vi "Wait on Read Loop.vi"(8 "error in (no error)":errorcluster, 10 "Value":bool, 11 "Terminal in":refnum<class "Terminal.lvclass">) -> (0 "error out":errorcluster, 1 "Timed Out?":bool, 3 "Terminal out":refnum<class "Terminal.lvclass">)   [LabVIEW 2020, in "Terminal.lvlib" / "Terminal.lvclass"]
uses:
  Terminal.lvclass
  Terminal.lvclass/Terminal.ctl
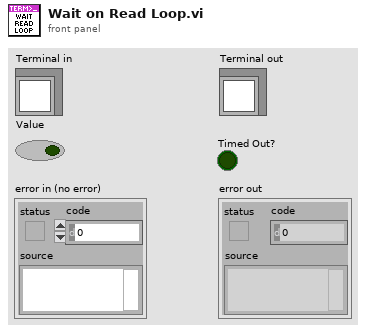
[diagram p1: front panel]
types:
  T1 = typedef "Terminal.lvlib/Terminal.lvclass/Ref Data.ctl" = cluster{"Connection":refnum<class "Connection.lvclass">, "Read Loop Running":bool, "Parse State":T2, "Terminal Options":T7, "Font Metrics":T10, "Scroll":i32, "Close Read Loop":bool}
  T2 = typedef "Terminal.lvlib/Terminal.lvclass/Parse State.ctl" = cluster{"Buffer State":T3, "Cursor":T4, "Attributes":T6}
  T3 = typedef "Terminal.lvlib/Terminal.lvclass/Buffer State.ctl" = cluster{"Sequence":string, "ESC":bool, "Alt Buf":bool}
  T4 = typedef "Terminal.lvlib/Terminal.lvclass/Cursor.ctl" = cluster{"Cur":T5, "Saved":T5}
  T5 = typedef "Terminal.lvlib/Terminal.lvclass/Position.ctl" = cluster{"Row":i32, "Col":i32}
  T6 = typedef "Terminal.lvlib/Text Attributes.ctl" = cluster{"FG":u32, "BG":u32, "Bold":bool, "Italic":bool, "Underline":bool, "Strike":bool, "Inverse":bool}
  T7 = typedef "Terminal.lvlib/Terminal Options.ctl" = cluster{"Implied CR with LF":bool, "Local Echo":bool, "Tab Width":i32, "Color Scheme":T8, "Default FG":T9, "Default BG":T9, "History Length":i32, "Font Face":string, "Font Size":i16, "Rows":i32, "Cols":i32}
  T8 = typedef "Terminal.lvlib/Color Scheme.ctl" = cluster{"Black":u32, "Red":u32, "Green":u32, "Yellow":u32, "Blue":u32, "Magenta":u32, "Cyan":u32, "White":u32, "Bright Black":u32, "Bright Red":u32, "Bright Green":u32, "Bright Yellow":u32, "Bright Blue":u32, "Bright Magenta":u32, "Bright Cyan":u32, "Bright White":u32}
  T9 = typedef "Terminal.lvlib/Color.ctl" = i8
  T10 = typedef "Terminal.lvlib/Terminal.lvclass/Font Metrics.ctl" = cluster{"Width":i16, "Height":i16}
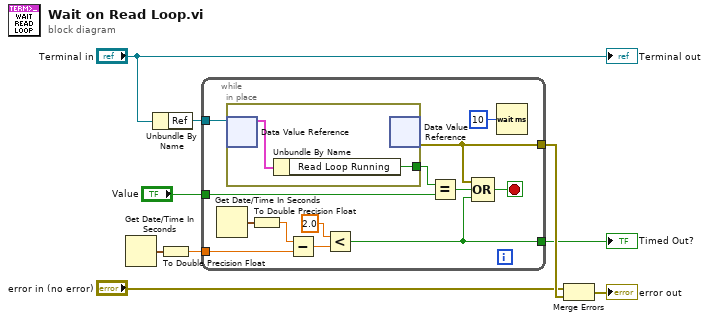
[diagram p0: block diagram]
diagram:
  n1 = Get Date/Time In Seconds() -> (seconds since 1Jan1904=w4:timestamp)
  n2 = Unbundle By Name("Terminal in") -> ("Ref"=w6:refnum<data-value>)
  n3 = To Double Precision Float(number=w4) -> (double precision float=w3:dbl)
  n4 = while {
    tunnel: w6 -> [w22]
    tunnel: "Value" -> [w20]
    tunnel: w3 -> [w16]
    tunnel: [w12] -> w2
    tunnel: [w10] -> w9
    stop <- w11 stop-if-true
    n5 = Get Date/Time In Seconds() -> (seconds since 1Jan1904=w17:timestamp)
    n6 = in-place {
      in-place-border: [w23] -> w19
      n7 = in-place-dvr #1(w22) -> (w24:T1)  [unwired: 1 out]
      n8 = Unbundle By Name(w24) -> ("Read Loop Running"=w23:bool)
      n9 = in-place-dvr #1() -> (w10:errorcluster)  [unwired: 1 in, 1 out]
    }
    n10 = To Double Precision Float(number=w17) -> (double precision float=w15:dbl)
    n11 = Subtract(x=w15, y=w16) -> (x-y=w14:dbl)
    n12 = Less?(x=2.0, y=w14) -> (x < y?=w12:bool)
    n13 = Equal?(x=w19, y=w20) -> (x = y?=w18:bool)
    n14 = Compound Arithmetic op=OR(w10, w18, w12) -> (w11:bool)
    n15 = Wait (ms)(milliseconds to wait=u32 10) -> ()  [unwired: 1 out]
  }
  "Timed Out?" <- w2
  n16 = Merge Errors("error in (no error)", w9) -> (→"error out":errorcluster)
  "Terminal out" <- "Terminal in"
